vi "SPCGetTimeScaleFromSETfile.vi"(8 "error in":errorcluster, 11 "setFile":path=path "C:/Users/jannis/Desktop/SPC file example/v1.set") -> (0 "error out":errorcluster, 1 "tac_gain":i16, 2 "tac_range":dbl, 3 "TimeAxisMultiplicator":dbl, 4 "adc_resolution":i16, 5 "bhfile_header":T2 {"chksum" format="x%x"; "header_valid" format="x%x"}, 6 "SetUp":string, 7 "FileInfo":string)   [LabVIEW 2019]
doc: "This VI demonstrates how parameters can be retrieved from a SDT- or SET-file's SetUp-block.\nSee also a different approach at \\Public\\Data\\SDT Files\\SDT_ReadSetUpBlock.vi.\nFor a description of the *.set file format see: SPC_data_file_structure.h\n\ninfo@becker-hickl.com"
uses:
  SPC_Controls/bhfile_header.ctl
  SPC_Controls/BHModuleType.ctl
panel:
  out "SetUpLength":i32
  out "ModuleSubtype":i16
  out "BHModuleType":T1=32 format="x%x" items=["SPC-130"=32, "SPC-600"=33, "SPC-630"=34, "SPC-700"=35, "SPC-730"=36, "SPC-830"=37, "SPC-140"=38, "SPC-930"=39, "SPC-150"=40, "DPC-230"=41, "SPC-130EM"=42, "SPC-160"=43, "SPC-150N"=46, "SPC-150NX"=128, "SPC-160X"=129, "SPC-160PCIE"=130, "SPC-130EMN"=131, "SPC-180N"=132, "SPC-180NX"=133, "SPC-180NXX"=134, "SPC-180N-USB"=135, "SPC-130IN"=136, "SPC-130INX"=137, "SPC-130INXX"=138, "SPC-QC-104"=139, "Simulation"=-1]
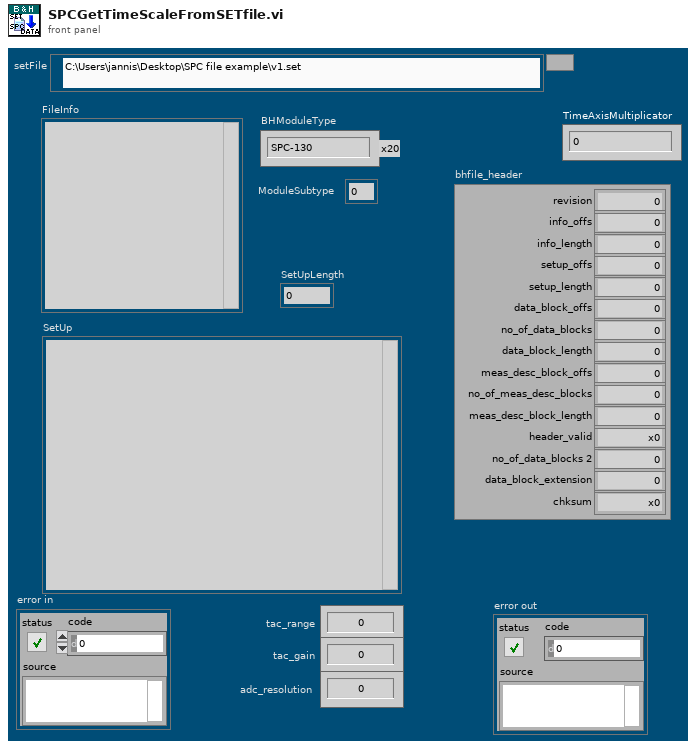
[diagram p1: front panel]
types:
  T1 = typedef "BHModuleType.ctl" = i16
  T2 = typedef "bhfile_header.ctl" = cluster{"revision":i16, "info_offs":i32, "info_length":i16, "setup_offs":i32, "setup_length":u16, "data_block_offs":i32, "no_of_data_blocks":i16, "data_block_length":u32, "meas_desc_block_offs":i32, "no_of_meas_desc_blocks":i16, "meas_desc_block_length":i16, "header_valid":u16, "no_of_data_blocks 2":u32, "data_block_extension":u16, "chksum":u16}
  T3 = enum16{"big-endian, network order", "native, host order", "little-endian"}
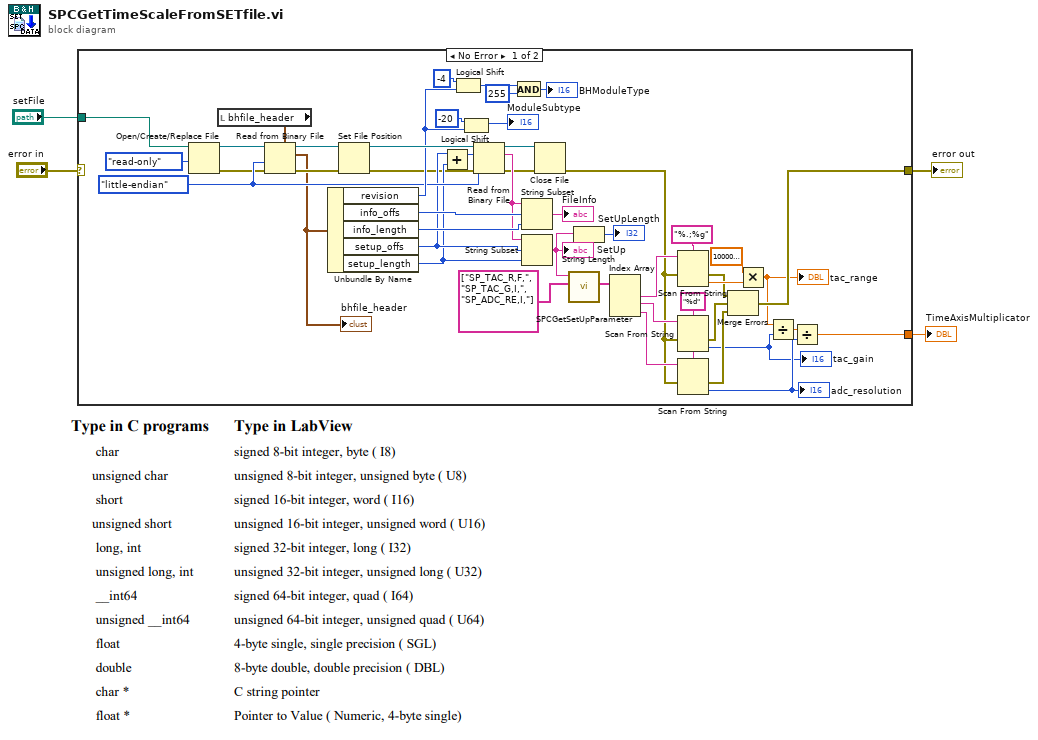
[diagram p0: block diagram]
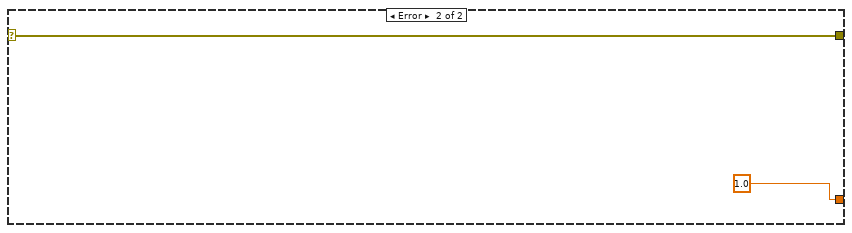
[diagram p2: hidden frame]
diagram:
  n1 = case shown="No Error" "error in" {
    selector: "error in" -> [_ w54]
    tunnel: "setFile" -> [w43 _]
    tunnel: [w10 w54] -> w3
    tunnel: [w17 1.0] -> w1
    frame No Error {
      w19 = "%d" ("format string")
      w37 = T3."little-endian" ("byte order (0:big-endian, network order)")
      n2 = Open/Create/Replace File(file path (use dialog)=w43, access (0:read/write)=enum16{"read/write", "read-only", "write-only"}."read-only") -> (refnum out=w42:refnum<file>, error out=w31:errorcluster)  [unwired: 4 in, 1 out]
      n3 = local read "bhfile_header"() -> (w5:T2)
      n4 = Read from Binary File(5:w5, 8:w31, 9:w37, 11:w42) -> (0:w30:errorcluster, 2:w6:T2, 3:w41:refnum<file>)  [unwired: 2 in, 1 out]
      "bhfile_header" <- w6
      n5 = Unbundle By Name(w6) -> ("revision"=w38:i16, "info_offs"=w46:i32, "info_length"=w45:i16, "setup_offs"=w35:i32, "setup_length"=w34:u16)
      n6 = Set File Position(refnum=w41, error in=w30) -> (refnum out=w40:refnum<file>, error out=w29:errorcluster)  [unwired: 2 in]
      n7 = Add(x=w35, y=w34) -> (x+y=w39:i32)
      n8 = Logical Shift(y=i16 -4, x=w38) -> (x << y=w50:i16)
      n9 = Logical Shift(y=i16 -20, x=w38) -> (x << y=→"ModuleSubtype":i16)
      n10 = Read from Binary File(8:w29, 9:w37, 10:w39, 11:w40) -> (0:w28:errorcluster, 2:w36:string, 3:w27:refnum<file>)  [unwired: 2 in, 1 out]
      n11 = And(x=w50, y=i16 255) -> (x .and. y?=→"BHModuleType":i16)
      n12 = String Subset(string=w36, offset (0)=w46, length (rest)=w45) -> (substring=→"FileInfo":string)
      n13 = String Subset(string=w36, offset (0)=w35, length (rest)=w34) -> (substring=w26:string)
      "SetUp" <- w26
      n14 = Close File(refnum=w27, error in=w28) -> (error out=w11:errorcluster)  [unwired: 1 out]
      n15 = call "SPCGetSetUpParameter.vi"("Key"=string[] ["SP_TAC_R,F,", "SP_TAC_G,I,", "SP_ADC_RE,I,"], "SetupString"=w26) -> ("Value"=w24:string[])  [unwired: 9 in]
      n16 = String Length(string=w26) -> (length=→"SetUpLength":i32)
      n17 = Index Array(array=w24) -> (element #1=w23:string, element #2=w21:string, element #3=w20:string)  [unwired: 3 in]
      n18 = Scan From String(format string="%.;%g", input string=w23, error in=w11) -> (error out=w14:errorcluster, output 1=w16:dbl)  [unwired: 2 in, 2 out]
      n19 = Scan From String(format string=w19, input string=w21, error in=w11) -> (error out=w13:errorcluster, output 1=w7:i16)  [unwired: 2 in, 2 out]
      "tac_gain" <- w7
      n20 = Scan From String(format string=w19, input string=w20, error in=w11) -> (error out=w12:errorcluster, output 1=w8:i16)  [unwired: 2 in, 2 out]
      "adc_resolution" <- w8
      n21 = Merge Errors(w14, w13, w12) -> (w10:errorcluster)
      n22 = Multiply(x=1000000000.0 ("y"), y=w16) -> (x*y=w9:dbl)
      "tac_range" <- w9
      n23 = Divide(x=w9, y=w7) -> (x/y=w18:dbl)
      n24 = Divide(x=w18, y=w8) -> (x/y=w17:dbl)
    }
    frame Error {
    }
  }
  "error out" <- w3
  "TimeAxisMultiplicator" <- w1
